vi "Register for Remote Events.vi"(8 "error in (no error)":errorcluster, 11 "Event Reporter Module in":refnum<class "Event Reporter Module.lvclass">) -> (0 "error out":errorcluster, 3 "Event Reporter Module out":refnum<class "Event Reporter Module.lvclass">)   [LabVIEW 2020, in "Volatus.lvlib" / "Event Reporter Module.lvclass"]
uses:
  Event Reporter Module.lvclass
  C:/dev/lv20CE/relink/lv-volatus/Volatus/Module/Module.lvclass
  Message Registration.ctl
  Event Reporter Module.lvclass/Event Reporter Module.ctl
  Module/Module.lvclass
  Volatus.lvlib
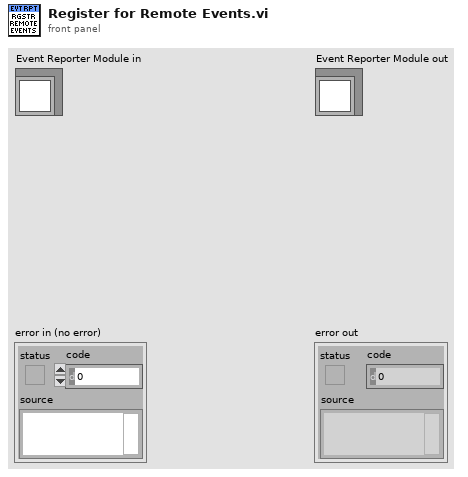
[diagram p1: front panel]
types:
  T1 = typedef "Volatus.lvlib/Message Registration.ctl" = cluster{"Message Type":string, "Message ID":string}
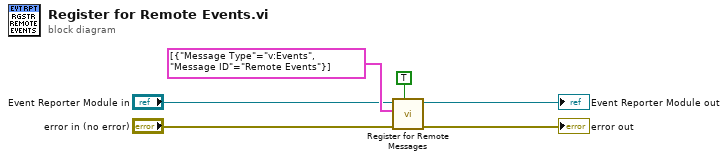
[diagram p0: block diagram]
diagram:
  n1 = call "Register for Remote Messages.vi"("Force (F)"=TRUE, "error in (no error)"="error in (no error)", "Messages"=T1[] [{"Message Type"="v:Events", "Message ID"="Remote Events"}], "Module in"="Event Reporter Module in") -> ("error out"=→"error out":errorcluster, "Module out"=→"Event Reporter Module out":refnum<class "Event Reporter Module.lvclass">)  [unwired: 6 in]
